vi "GD_GWID3F_info.vi"(7 "glue_id":string, 8 "error in (no error)":errorcluster, 10 "glue_1":sgl, 11 "DBlink":string="Driver={ODBC Driver 17 for SQL Server};Server=localhost\\SQLEXPRESS;Database=ZDX201;UID=labview;PWD=Dsa@54137926") -> (0 "error out":errorcluster)   [LabVIEW 2019]
uses:
  <vilib>/addons/database/Auxilliary.llb/DB Tools Format Datetime String (Time Stamp).vi
  <vilib>/addons/database/Connection.llb/DB Tools Open Connec (String).vi
  <vilib>/addons/database/NI_Database_API.lvlib
panel:
  out "Command 2":string="WHERE [id]=0"
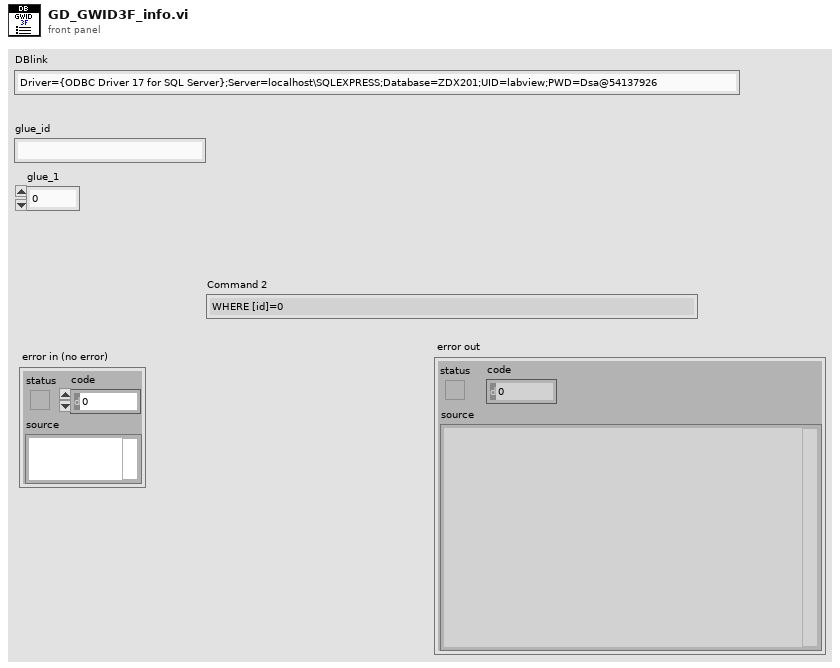
[diagram p1: front panel]
types:
  T1 = cluster{"glue_1":sgl, "update_time":timestamp, "time_finish_1":timestamp}
  T2 = typedef "NI_Database_API.lvlib/Conn ObjectReference.ctl" = refnum<k1>
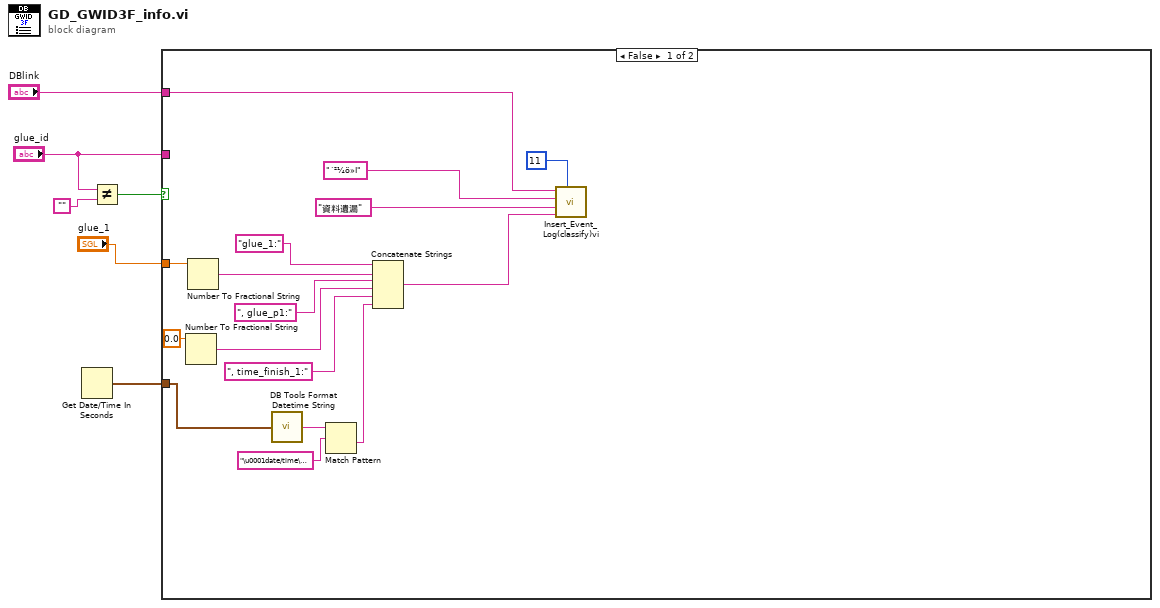
[diagram p0: block diagram]
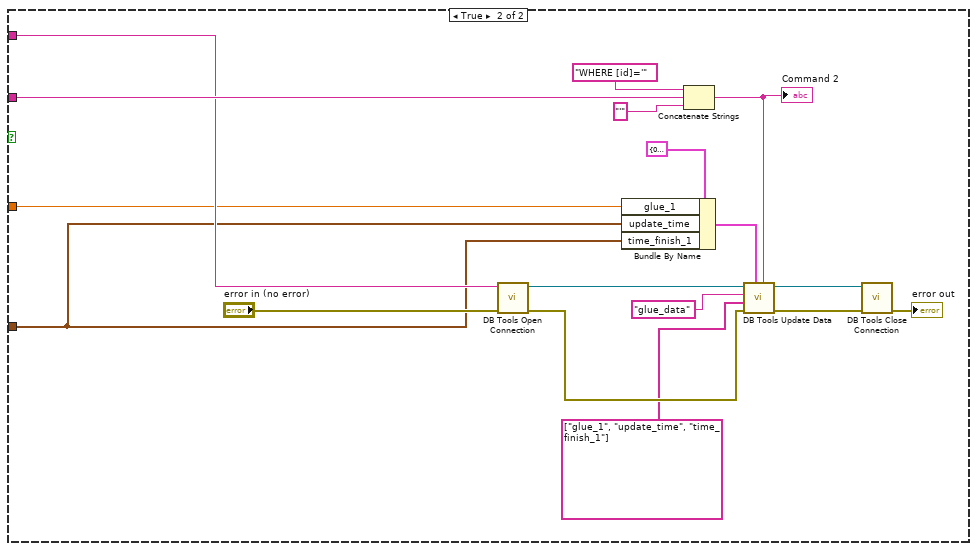
[diagram p2: hidden frame]
diagram:
  n1 = Get Date/Time In Seconds() -> (seconds since 1Jan1904=w1:timestamp)
  n2 = Not Equal?(x="glue_id", y="") -> (x != y?=w6:bool)
  n3 = case shown="False" w6 {
    tunnel: "glue_id" -> [_ w26]
    tunnel: "DBlink" -> [w22 w25]
    tunnel: "glue_1" -> [w17 w24]
    tunnel: w1 -> [w11 w23]
    frame False {
      n4 = Number To Fractional String(number=0.0) -> (F-format string=w13:string)  [unwired: 3 in]
      n5 = Number To Fractional String(number=w17) -> (F-format string=w15:string)  [unwired: 3 in]
      n6 = call-poly <vilib>:"DB Tools Format Datetime String.vi"("time stamp"=w11) -> ("date/time string"=w18:string)
      n7 = Match Pattern(string=w18, regular expression="\u0001date/time\u0001" ("search string")) -> (after substring=w10:string)  [unwired: 1 in, 3 out]
      n8 = Concatenate Strings("glue_1:", w15, ", glue_p1:", w13, ", time_finish_1:", w10) -> (w9:string)
      n9 = call "Insert_Event_Log(classify)vi.vi"("classify"=i16 11, "data"=w9, "message"="資料遺漏", "id"="´²¼ö»I", "DBlink"=w22) -> ()  [unwired: 6 in, 1 out]
    }
    frame True {
      n10 = call-poly <vilib>:"DB Tools Open Connection.vi"("error in (no error)"="error in (no error)", "connection information"=w25) -> ("error out"=w38:errorcluster, "connection reference"=w29:T2)  [unwired: 6 in]
      n11 = Bundle By Name(cluster=T1 {"glue_1"=0.0, "update_time"=timestamp(0 s since 1904-01-01), "time_finish_1"=timestamp(0 s since 1904-01-01)}, "glue_1"=w24, "update_time"=w23, "time_finish_1"=w23) -> (w30:T1)
      n12 = Concatenate Strings("WHERE [id]='", w26, "'" ("string")) -> (w32:string)
      "Command 2" <- w32
      n13 = call <vilib>:"DB Tools Update Data.vi"("condition"=w32, "data"=w30, "error in (no error)"=w38, "columns"=string[] ["glue_1", "update_time", "time_finish_1"], "table"="glue_data", "connection reference"=w29) -> ("error out"=w39:errorcluster, "connection reference out"=w37:T2)  [unwired: 4 in]
      n14 = call <vilib>:"DB Tools Close Connection.vi"("error in (no error)"=w39, "connection reference"=w37) -> ("error out"=→"error out":errorcluster)  [unwired: 5 in]
    }
  }
